vi "OAT Remove Slow Roll Error (Single Channel).vi"(6 "phase setting":T1, 7 "reset? (True)":bool=TRUE, 8 "error in (no error)":errorcluster, 9 "slow roll vectors":cdb[](array[numeric]) format="%.2f", 10 "phase lags":cluster{"X":dbl[], "Y":dbl[]}[](array[cluster]) {"Y" format="%.2f"; "X" format="%.2f"}, 11 "magnitudes (RMS)":cluster{"X":dbl[], "Y":dbl[]}[](array[cluster]) {"Y" format="%.2f"; "X" format="%.2f"}) -> (0 "error out":errorcluster, 1 "actual slow roll vectors":cdb[](array[numeric]) format="%.2f", 2 "compensated phase lags":cluster{"X":dbl[], "Y":dbl[]}[](array[cluster]) {"Y" format="%.2f"; "X" format="%.2f"}, 3 "compensated magnitudes (RMS)":cluster{"X":dbl[], "Y":dbl[]}[](array[cluster]) {"Y" format="%.2f"; "X" format="%.2f"})   [LabVIEW 2017]
doc: "Performs run out compensation for proximity probe signals. This vi receives <B>magnitudes (RMS)</B> and <B>phase lags</B> from the order tracking vis and the <B>slow roll vectors</B> of the same orders.It removes the slow roll errors by subtracting the <B>slow roll vectors</B> from the corresponding <B>magnitudes (RMS)</B> and <B>phase lags</B>."
uses:
  <vilib>/addons/Sound and Vibration/Order Analysis/Misc/OAT Convert Phase (1 channel).vi
  <vilib>/Analysis/NI_AALPro.lvlib
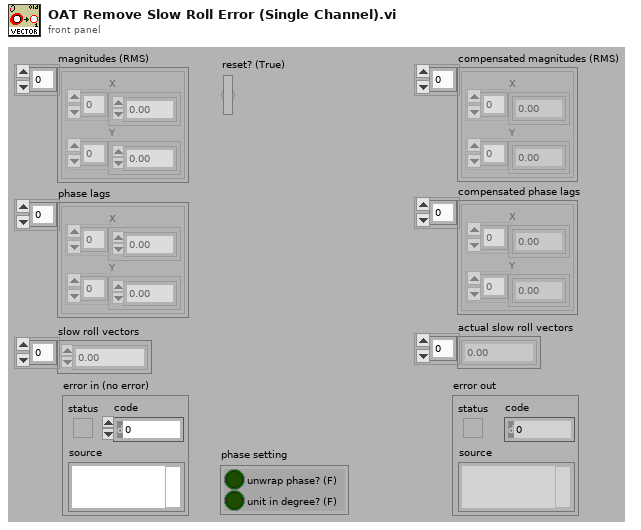
[diagram p1: front panel]
types:
  T1 = cluster{"unwrap phase? (F)":bool, "unit in degree? (F)":bool}
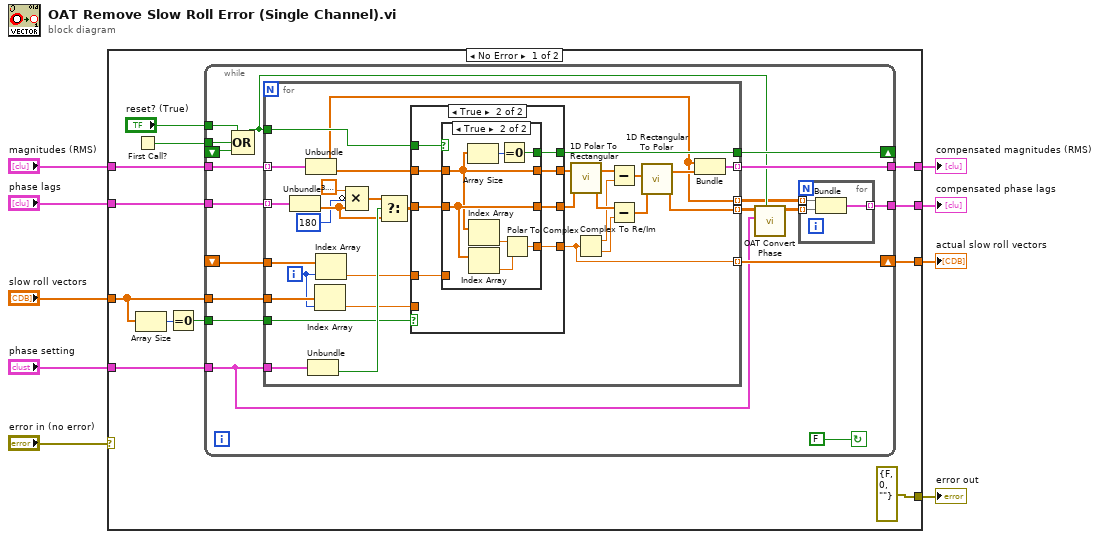
[diagram p0: block diagram]
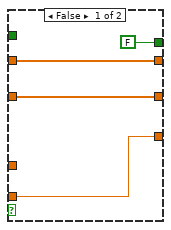
[diagram p2: hidden frame]
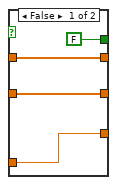
[diagram p3: hidden frame]
diagram:
  n1 = case shown="No Error" "error in (no error)" {
    selector: "error in (no error)" -> [_ w100]
    tunnel: "magnitudes (RMS)" -> [w15 w99]
    tunnel: "phase lags" -> [w21 w98]
    tunnel: "slow roll vectors" -> [w12 w97]
    tunnel: [w20 w99] -> w6
    tunnel: [w19 w98] -> w5
    tunnel: [errorcluster {"status"=FALSE, "code"=0, "source"=""} ("error IO") w100] -> w3
    tunnel: [w17 w97] -> w2
    tunnel: "phase setting" -> [w14 _]
    frame No Error {
      n2 = First Call?() -> (First Call?: T/F=w11:bool)
      n3 = Array Size(array=w12) -> (size(s)=w16:i32)
      n4 = Equal To 0?(x=w16) -> (x = 0?=w13:bool)
      n5 = while {
        tunnel: w15 -> [w37]
        tunnel: w21 -> [w36]
        tunnel: [w39] -> w20
        tunnel: [w22] -> w19
        shift-right: [w35] -> w17
        shift-left: _ -> [w34]
        tunnel: w14 -> [w25]
        tunnel: w13 -> [w33]
        tunnel: w12 -> [w32]
        shift-right: [w31] -> _
        shift-left: _ -> [w30]
        tunnel: w11 -> [w29]
        tunnel: "reset? (True)" -> [w28]
        stop <- FALSE continue-if-true
        n6 = Compound Arithmetic op=OR(w28, w29, w30) -> (w26:bool)
        n7 = for {
          tunnel: w37 -> [w73] mode=indexing
          tunnel: w36 -> [w72] mode=indexing
          tunnel: [w71] -> w39 mode=indexing
          tunnel: [w56] -> w35 mode=indexing
          tunnel: w34 -> [w55]
          tunnel: w26 -> [w45]
          tunnel: w25 -> [w59]
          tunnel: w33 -> [w51]
          tunnel: w32 -> [w53]
          tunnel: [w49] -> w31
          tunnel: [w44] -> w27 mode=indexing
          tunnel: [w43] -> w23 mode=indexing
          i -> [w52]
          n8 = Unbundle(w72) -> ("Y"=w48:dbl[])  [unwired: 1 out]
          n9 = Unbundle(w73) -> ("X"=w43:dbl[], "Y"=w70:dbl[])
          n10 = Unbundle(w59) -> ("unit in degree? (F)"=w62:bool)  [unwired: 1 out]
          n11 = Index Array(array=w53, index=w52) -> (element=w50:cdb)
          n12 = Index Array(array=w55, index=w52) -> (element=w54:cdb)
          n13 = Compound Arithmetic op=MULTIPLY(3.141592653589793, invert 180, w48) -> (w60:dbl[])
          n14 = Select(t=w60, s=w62, f=w48) -> (s? t:f=w61:dbl[])
          n15 = case shown="True" w51 {
            tunnel: w45 -> [_ w85]
            tunnel: w70 -> [w75 w84]
            tunnel: [w75 w83] -> w69
            tunnel: [w76 w82] -> w68
            tunnel: w61 -> [w76 w81]
            tunnel: [w77 w80] -> w56
            tunnel: w54 -> [_ w79]
            tunnel: w50 -> [w77 _]
            tunnel: [FALSE w78] -> w49
            frame False {
            }
            frame True {
              n16 = case shown="True" w85 {
                tunnel: w84 -> [w88 w92]
                tunnel: [w89 w93] -> w80
                tunnel: w81 -> [w87 w96]
                tunnel: w79 -> [w89 _]
                tunnel: [w88 w92] -> w83
                tunnel: [w87 w96] -> w82
                tunnel: [FALSE w90] -> w78
                frame False {
                }
                frame True {
                  n17 = Array Size(array=w92) -> (size(s)=w91:i32)
                  n18 = Index Array(array=w92) -> (element=w95:dbl)  [unwired: 1 in]
                  n19 = Index Array(array=w96) -> (element=w94:dbl)  [unwired: 1 in]
                  n20 = Equal To 0?(x=w91) -> (x = 0?=w90:bool)
                  n21 = Polar To Complex(1:w94, 2:w95) -> (0:w93:cdb)
                }
              }
            }
          }
          n22 = call <vilib>:"1D Polar To Rectangular.vi"("Magnitude"=w69, "Phase"=w68) -> ("X"=w67:dbl[], "Y"=w66:dbl[])  [unwired: 1 out]
          n23 = Complex To Re/Im(x + iy=w56) -> (x=w58:dbl, y=w57:dbl)
          n24 = Subtract(x=w67, y=w58) -> (x-y=w65:dbl[])
          n25 = Subtract(x=w66, y=w57) -> (x-y=w64:dbl[])
          n26 = call <vilib>:"1D Rectangular To Polar.vi"("X"=w65, "Y"=w64) -> ("Magnitude"=w63:dbl[], "Phase"=w44:dbl[])  [unwired: 1 out]
          n27 = Bundle("X"=w43, "Magnitude"=w63) -> (w71:cluster{"X":dbl[], "Magnitude":dbl[]})  [unwired: 1 in]
        }
        n28 = call-poly <vilib>:"OAT Convert Phase.vi"("reset (TRUE)"=w26, "desired phase setting"=w25, "phase in (rad)"=w27) -> ("phase out"=w24:dbl[][])  [unwired: 8 in]
        n29 = for {
          tunnel: w24 -> [w41] mode=indexing
          tunnel: w23 -> [w42] mode=indexing
          tunnel: [w40] -> w22 mode=indexing
          n30 = Bundle("X"=w42, "phase out"=w41) -> (w40:cluster{"X":dbl[], "phase out":dbl[]})  [unwired: 1 in]
        }
      }
    }
    frame Error {
    }
  }
  "error out" <- w3
  "compensated magnitudes (RMS)" <- w6
  "compensated phase lags" <- w5
  "actual slow roll vectors" <- w2
